vi "Actor Core.vi"(8 "error in":errorcluster, 11 "My Application":refnum<class "LVAutomationListener.lvclass">) -> (0 "error out":errorcluster, 3 "Actor out":refnum<class "Actor.lvclass">)   [LabVIEW 2013, in "LVAutomationListener.lvlib" / "LVAutomationListener.lvclass"]
doc: "This is Actor Core.vi, the main message handling loop for Actors. An actor usually just sits in this loop and processes messages as they arrive. Any error returned by the message Do.vi call will stop the loop, with error code 43 as the canonical signal to stop with no error sent to caller. Descendants may override that in Handle Error.vi."
uses:
  LVAutomationListener.lvclass
  <vilib>/ActorFramework/Actor/Actor.lvclass
  <vilib>/ActorFramework/Actor/Actor.lvclass/Actor.ctl
  <vilib>/ActorFramework/Message Enqueuer/Message Enqueuer.lvclass/Message Enqueuer.ctl
  LVAutomationListener.lvclass/LVAutomationListener.ctl
  <vilib>/ActorFramework/Message Enqueuer/Init from Existing Queue.vi
  <vilib>/ActorFramework/Message Enqueuer/Enqueue.vi
  <vilib>/ActorFramework/Message Priority Queue/Priority Enqueue.vi
  <vilib>/ActorFramework/Message Enqueuer/Message Enqueuer.lvclass
  msgs/Abort Msg/Abort Msg.lvclass
  tWorkerController/tWorkerController/tWorkerController.lvclass
panel:
  out "Listener Status":string
  in  "stop signal":bool
  in  "Stop":bool
  # "Controller"
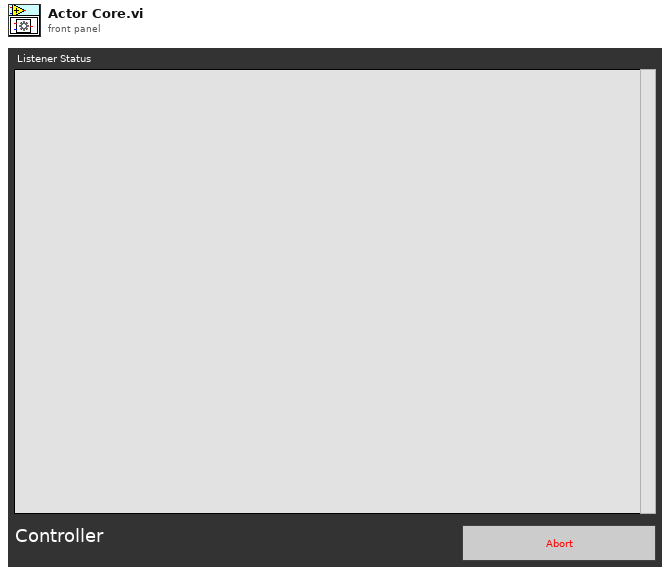
[diagram p1: front panel]
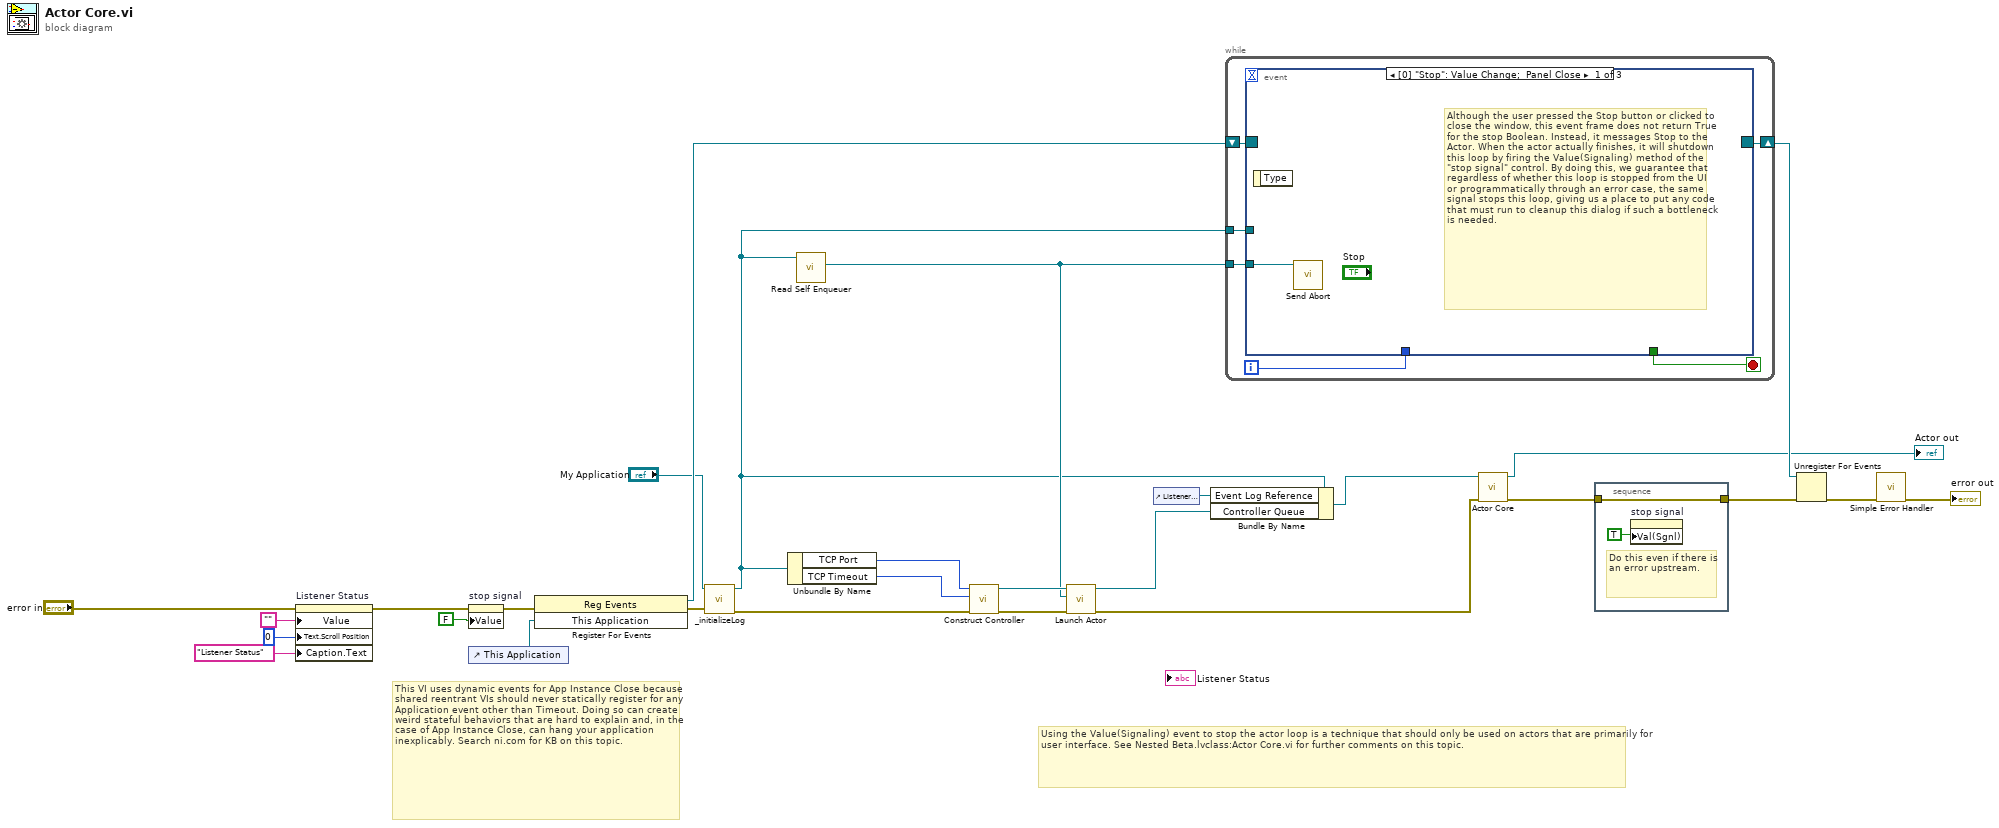
[diagram p0: block diagram]
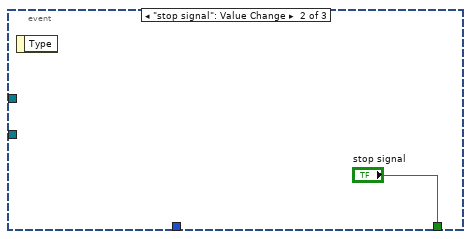
[diagram p2: hidden frame]
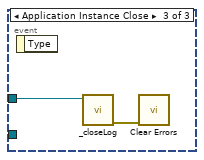
[diagram p3: hidden frame]
diagram:
  # "This VI uses dynamic events for App Instance Close because shared reentrant VIs should never statically register for any Application event other than Timeout. Doing so can create weird stateful behaviors that are hard to explain and, in the case of App Instance Close, can hang your application inexplicably. Search ni.com for KB on this topic."
  # "Using the Value(Signaling) event to stop the actor loop is a technique that should only be used on actors that are primarily for user interface. See Nested Beta.lvclass:Actor Core.vi for further comments on this topic."
  n1 = property on="Listener Status" class="Str"(error in="error in", "Value"="", "Text.Scroll Position"=u32 0, "Caption.Text"="Listener Status" ("Unlocalized")) -> (error out=w18:errorcluster)  [unwired: 1 in, 1 out]
  n2 = property on="stop signal" class="Bool (strict)"(error in=w18, "Value"=FALSE ("stop")) -> (error out=w25:errorcluster)  [unwired: 1 in, 1 out]
  n3 = control-ref of="This Application"() -> (w24:refnum<vi>)
  n4 = register-events(error in=w25, w24) -> (reference out=w27:refnum<event-registration>, error out=w12:errorcluster)  [unwired: 1 in]
  n5 = call "_initializeLog.vi"("error in (no error)"=w12, "SkynetCompiler in"="My Application") -> ("error out"=w9:errorcluster, "SkynetCompiler out"=w10:refnum<class "LVAutomationListener.lvclass">)  [unwired: 8 in]
  n6 = Unbundle By Name(w10) -> ("TCP Port"=w17:u16, "TCP Timeout"=w16:i32)
  n7 = call <vilib>:"Read Self Enqueuer.vi"("Actor"=w10) -> ("Self Enqueuer"=w13:refnum<class "Message Enqueuer.lvclass">)  [unwired: 10 in]
  n8 = call "Construct Controller.vi"("error in (no error)"=w9, "TCP Timeout"=w16, "TCP Port"=w17) -> ("error out"=w15:errorcluster, "tWorkerController out"=w14:refnum<class "tWorkerController.lvclass">)  [unwired: 7 in]
  n9 = call <vilib>:"Launch Actor.vi"("error in (no error)"=w15, "Actor-to-Caller Enqueuer"=w13, "Actor"=w14) -> ("error out"=w1:errorcluster, "Caller-To-Actor Enqueuer"=w3:refnum<class "Message Enqueuer.lvclass">)  [unwired: 7 in]
  n10 = control-ref of="Listener Status"() -> (w23:refnum<vi>)
  n11 = Bundle By Name(cluster=w10, "Event Log Reference"=w23, "Controller Queue"=w3) -> (w2:refnum<class "LVAutomationListener.lvclass">)
  n12 = while {
    tunnel: w13 -> [w34]
    shift-right: [w30] -> w26
    shift-left: w27 -> [w31]
    tunnel: w10 -> [w29]
    i -> [w32]
    stop <- w33 stop-if-true
    n13 = event shown="[0] \"Stop\": Value Change;  Panel Close" {
      selector: w31 -> [_ _ _]
      dyn-events: [_ _ _] -> w30
      timeout: _ -> [_ _ _]
      tunnel: w34 -> [w35 _ _]
      tunnel: [_ "stop signal" _] -> w33
      tunnel: w32 -> [_ _ _]
      tunnel: w29 -> [_ _ w38]
      event "Stop": Value Change; Panel Close {
        # "Although the user pressed the Stop button or clicked to close the window, this event frame does not return True for the stop Boolean. Instead, it messages Stop to the Actor. When the actor actually finishes, it will shutdown this loop by firing the Value(Signaling) method of the \"stop signal\" control. By doing this, we guarantee that regardless of whether this loop is stopped from the UI or programmatically through an error case, the same signal stops this loop, giving us a place to put any code that must run to cleanup this dialog if such a bottleneck is needed."
        n14 = event-data() -> ()  [unwired: 1 in, 1 out]
        n15 = call "Send Abort.vi"("Message Enqueuer"=w35) -> ()  [unwired: 9 in, 2 out]
      }
      event "stop signal": Value Change {
        n16 = event-data() -> ()  [unwired: 1 in, 1 out]
      }
      event Application Instance Close {
        n17 = event-data() -> ()  [unwired: 1 in, 1 out]
        n18 = call "_closeLog.vi"("SkynetCompiler in"=w38) -> ("error out"=w37:errorcluster)  [unwired: 9 in, 1 out]
        n19 = call <vilib>:"Clear Errors.vi"("error in (no error)"=w37) -> ()  [unwired: 6 in, 1 out]
      }
    }
  }
  n20 = call-parent "Actor Core.vi"("error in"=w1, "Actor in"=w2) -> ("error out"=w7:errorcluster, "Actor out"=→"Actor out":refnum<class "Actor.lvclass">)  [unwired: 8 in]
  n21 = stacked-sequence {
    tunnel: [w39] -> w8
    tunnel: w7 -> [w39]
    frame #0 {
      # "Do this even if there is an error upstream."
      n22 = property on="stop signal" class="Bool (strict)"("Val(Sgnl)"=TRUE ("stop")) -> ()  [unwired: 2 in, 2 out]
    }
  }
  n23 = Unregister For Events(event registration refnum=w26, error in=w8) -> (error out=w6:errorcluster)
  n24 = call <vilib>:"Simple Error Handler.vi"("error in (no error)"=w6) -> ("error out"=→"error out":errorcluster)  [unwired: 4 in, 4 out]
